vi "PWM In, Latched (subVI).vi"(2 "Latch":bool, 3 "Input":bool) -> (0 "High Period":u32, 1 "Low Period":u32)   [LabVIEW 2015]
doc: "This VI supports a PWM measurement application. It returns the most recent PWM measurement when the latch button is pressed."
uses:
  Instance           1 20Saved   PWM, Latched .vi
panel:
  # "This VI supports a PWM measurement application.  It returns the most recent PWM measurement when the latch button is pressed."
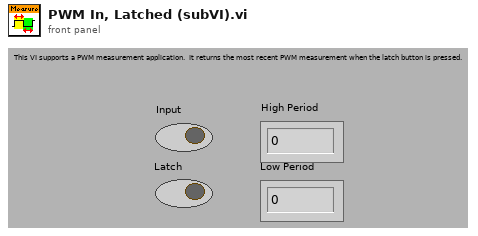
[diagram p1: front panel]
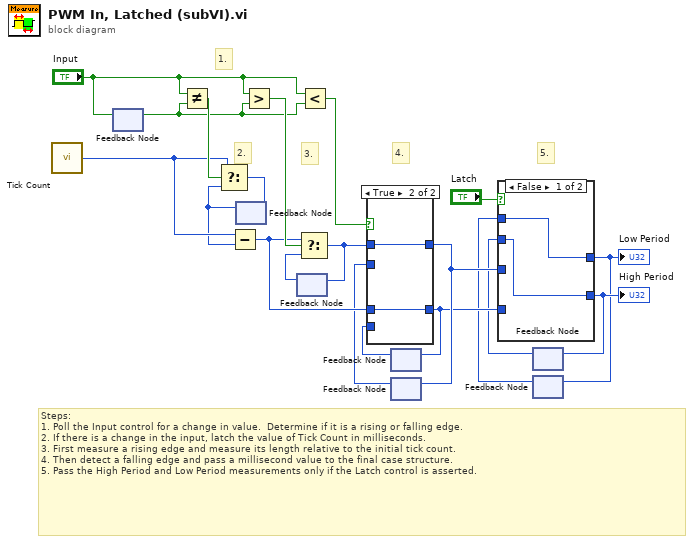
[diagram p0: block diagram]
diagram:
  # "5."
  # "4."
  # "3."
  # "2."
  # "1."
  # "Steps:\n1. Poll the Input control for a change in value.  Determine if it is a rising or falling edge.\n2. If there is a change in the input, latch the value of Tick Count in milliseconds.\n3. First measure a rising edge and measure its length relative to the initial tick count.\n4. Then detect a falling edge and pass a millisecond value to the final case structure.\n5. Pass the High Period and Low Period measurements only if the Latch control is asserted."
  n1 = call "Tick Count"() -> ("Tick Count(mSec)"=w16:u32)
  n2 = feedback-in #1("Input") -> ()
  n3 = feedback #1() -> (w14:bool)  [unwired: 1 out]
  n4 = Not Equal?(x="Input", y=w14) -> (x != y?=w20:bool)
  n5 = feedback #2() -> (w12:u32)  [unwired: 1 out]
  n6 = Select(t=w16, s=w20, f=w12) -> (s? t:f=w13:u32)
  n7 = Subtract(x=w16, y=w12) -> (x-y=w18:u32)
  n8 = feedback-in #2(w13) -> ()
  n9 = Greater?(x="Input", y=w14) -> (0:w19:bool)
  n10 = feedback #3() -> (w10:u32)  [unwired: 1 out]
  n11 = Select(t=w18, s=w19, f=w10) -> (s? t:f=w11:u32)
  n12 = feedback-in #3(w11) -> ()
  n13 = Less?(x="Input", y=w14) -> (x < y?=w17:bool)
  n14 = feedback #4() -> (w8:u32)  [unwired: 1 out]
  n15 = feedback #5() -> (w9:u32)  [unwired: 1 out]
  n16 = case shown="True" w17 {
    tunnel: w18 -> [_ w24]
    tunnel: [w21 w24] -> w6
    tunnel: w11 -> [_ w23]
    tunnel: [w22 w23] -> w7
    tunnel: w9 -> [w22 _]
    tunnel: w8 -> [w21 _]
    frame False {
    }
    frame True {
    }
  }
  n17 = feedback-in #4(w6) -> ()
  n18 = feedback-in #5(w7) -> ()
  n19 = feedback #6() -> (w4:u32)  [unwired: 1 out]
  n20 = feedback #7() -> (w5:u32)  [unwired: 1 out]
  n21 = case shown="False" "Latch" {
    tunnel: w6 -> [_ w28]
    tunnel: w7 -> [_ w27]
    tunnel: [w25 w27] -> w1
    tunnel: [w26 w28] -> w2
    tunnel: w5 -> [w25 _]
    tunnel: w4 -> [w26 _]
    frame False {
    }
    frame True {
    }
  }
  "Low Period" <- w1
  "High Period" <- w2
  n22 = feedback-in #6(w2) -> ()
  n23 = feedback-in #7(w1) -> ()
